vi "Switch status IO - Human Readable_3voltageamp.vi"(2 "PPMS      DR":bool=TRUE, 3 "Switch status":path=path "C:/LabView/PPMS basic VIs/Switch Status.txt") -> (0 "String":string="I-:2\nV1+:\nI+:1\nV-:5\n")   [LabVIEW 2011]
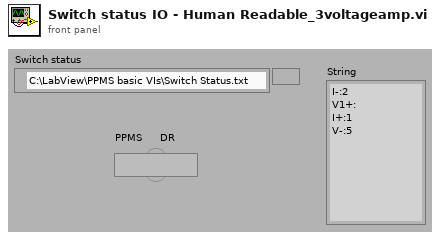
[diagram p1: front panel]
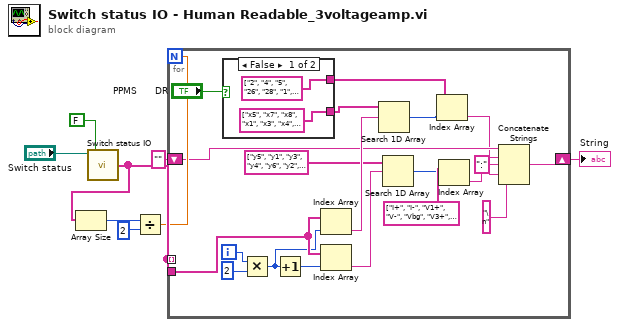
[diagram p0: block diagram]
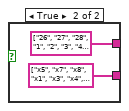
[diagram p2: hidden frame]
diagram:
  n1 = call "Switch status IO.vi"("Write: T\nRead: F"=FALSE ("Write: T\nRead: F"), "Path"="Switch status") -> ("String out"=w6:string[])  [unwired: 4 in]
  n2 = Array Size(array=w6) -> (size(s)=w3:i32)
  n3 = Divide(x=w3, y=2) -> (x/y=w5:dbl)
  n4 = for {
    N: w5 -> [_]
    tunnel: w6 -> [w28]
    tunnel: w6 -> [_] mode=indexing
    shift-right: [w15] -> w8
    shift-left: "" -> [w14]
    i -> [w26]
    n5 = case shown="False" "PPMS      DR" {
      tunnel: [string[] ["x5", "x7", "x8", "x1", "x3", "x4", "x2", "x6", "x11", "x12", "x10"] string[] ["x5", "x7", "x8", "x1", "x3", "x4", "x2", "x6"]] -> w23
      tunnel: [string[] ["2", "4", "5", "26", "28", "1", "27", "3", "24", "25", "6"] string[] ["26", "27", "28", "1", "2", "3", "4", "5"]] -> w21
      frame False {
      }
      frame True {
      }
    }
    n6 = Multiply(x=w26, y=2) -> (x*y=w24:i32)
    n7 = Increment(x=w24) -> (x+1=w27:i32)
    n8 = Index Array(array=w28, index=w24) -> (element=w22:string)
    n9 = Index Array(array=w28, index=w27) -> (element=w18:string)
    n10 = Search 1D Array(1D array=w23, element=w22) -> (index of element=w20:i32)  [unwired: 1 in]
    n11 = Search 1D Array(1D array=string[] ["y5", "y1", "y3", "y4", "y6", "y2", "y7", "y8"], element=w18) -> (index of element=w16:i32)  [unwired: 1 in]
    n12 = Index Array(array=w21, index=w20) -> (element=w11:string)
    n13 = Index Array(array=string[] ["I+", "I-", "V1+", "V-", "Vbg", "V3+", "V2+", "V2-"], index=w16) -> (element=w13:string)
    n14 = Concatenate Strings(w14, w13, ":" ("string"), w11, "\n" ("string")) -> (w15:string)
  }
  "String" <- w8
